vi "SBML_Functions.vi"(8 "error in (no error)":errorcluster, 11 "Input SBML File":string) -> (0 "error out":errorcluster, 1 "Fn Arg Cnt":string[](array[string]), 2 "Functions":string[][](table), 3 "FuncCnt":i32)   [LabVIEW 2014]
doc: "This VI extract the information of species present in SBML file. It takes the complete SBML file as input, and outputs: \nSp_Cnt --> How many species are there\nS_Id_Arr --> Array of species\nSp_Name --> Array containing the name of species\nSp_Init_Amnt --> Array containing the initial amount of species\n\nDesigned by HB\nhaba@dtu.dk"
panel:
  out "Math":string[](array[string])
  out "Name":string[](array[string])
  out "ID":string[](array[string])
  out "List of Functions":string
  # "Names"
  # "Initial Amount"
  # "ID"
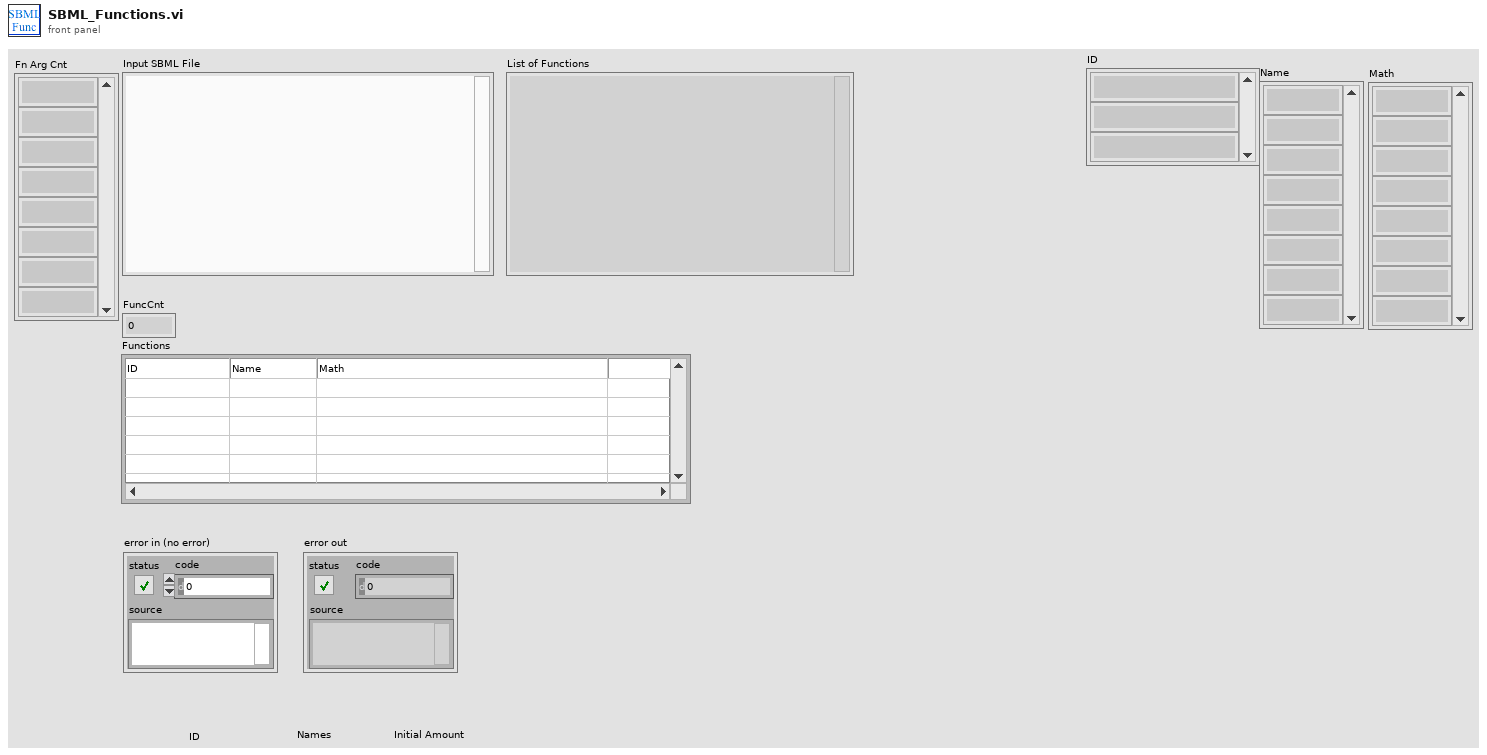
[diagram p1: front panel]
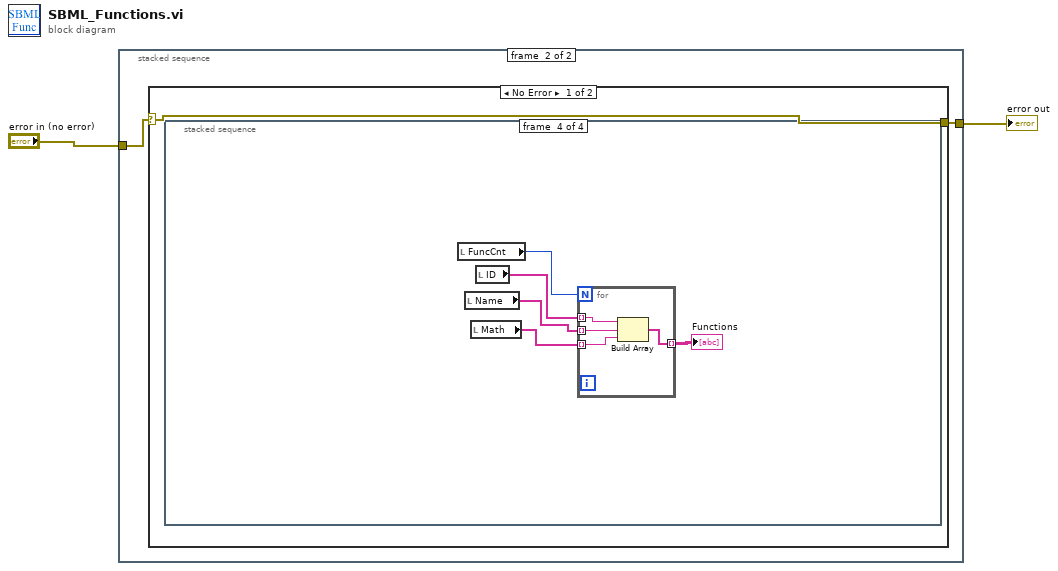
[diagram p0: block diagram]
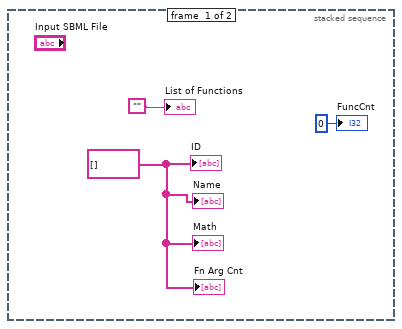
[diagram p2: hidden frame]
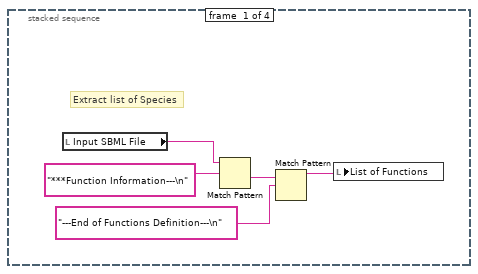
[diagram p3: hidden frame]
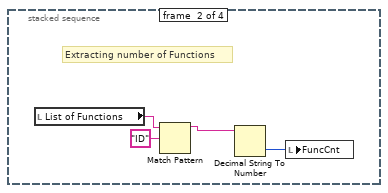
[diagram p4: hidden frame]
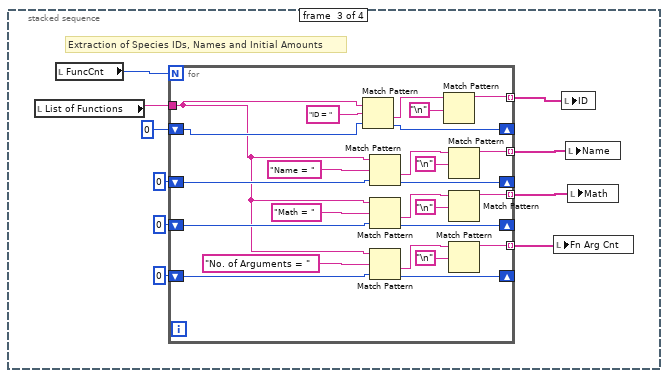
[diagram p5: hidden frame]
diagram:
  n1 = stacked-sequence {
    tunnel: "error in (no error)" -> [_ w6]
    tunnel: [_ w7] -> w1
    frame #0 {
      w3 = string[] [] ("Sp_Id_Arr")
      "List of Functions" <- "" ("Full SBML File")
      "FuncCnt" <- 0 ("Sp_cnt")
      "ID" <- w3
      "Name" <- w3
      "Math" <- w3
      "Fn Arg Cnt" <- w3
    }
    frame #1 {
      n2 = case shown="No Error" w6 {
        selector: w6 -> [w8 w62]
        tunnel: [w8 w62] -> w7
        frame No Error {
          n3 = stacked-sequence {
            frame #0 {
              # "Extract list of Species"
              n4 = local read "Input SBML File"() -> (w10:string)
              n5 = Match Pattern(string=w10, regular expression="***Function Information---\n") -> (after substring=w12:string)  [unwired: 1 in, 3 out]
              n6 = Match Pattern(string=w12, regular expression="---End of Functions Definition---\n") -> (before substring=w9:string)  [unwired: 1 in, 3 out]
              n7 = local write "List of Functions"(w9) -> ()
            }
            frame #1 {
              # "Extracting number of Functions"
              n8 = local read "List of Functions"() -> (w14:string)
              n9 = Match Pattern(string=w14, regular expression="ID") -> (before substring=w15:string)  [unwired: 1 in, 3 out]
              n10 = Decimal String To Number(string=w15) -> (number=w17:i32)  [unwired: 2 in, 1 out]
              n11 = local write "FuncCnt"(w17) -> ()
            }
            frame #2 {
              # "Extraction of Species IDs, Names and Initial Amounts"
              n12 = local read "List of Functions"() -> (w26:string)
              n13 = local read "FuncCnt"() -> (w25:i32)
              n14 = for {
                N: w25 -> [_]
                tunnel: w26 -> [w28]
                shift-right: [w41] -> _
                shift-left: 0 ("offset past match") -> [w42]
                tunnel: [w49] -> w24 mode=indexing
                shift-right: [w46] -> _
                shift-left: 0 ("offset past match") -> [w47]
                tunnel: [w48] -> w23 mode=indexing
                shift-right: [w37] -> _
                shift-left: 0 ("offset past match") -> [w36]
                tunnel: [w35] -> w20 mode=indexing
                shift-right: [w32] -> _
                shift-left: 0 ("offset past match") -> [w33]
                tunnel: [w34] -> w19 mode=indexing
                n15 = Match Pattern(string=w28, regular expression="ID = ", offset (0)=w42) -> (after substring=w50:string, offset past match=w41:i32)  [unwired: 2 out]
                n16 = Match Pattern(string=w28, regular expression="Name = ", offset (0)=w47) -> (after substring=w43:string, offset past match=w46:i32)  [unwired: 2 out]
                n17 = Match Pattern(string=w28, regular expression="Math = ", offset (0)=w36) -> (after substring=w40:string, offset past match=w37:i32)  [unwired: 2 out]
                n18 = Match Pattern(string=w28, regular expression="No. of Arguments = ", offset (0)=w33) -> (after substring=w29:string, offset past match=w32:i32)  [unwired: 2 out]
                n19 = Match Pattern(string=w50, regular expression="\n") -> (before substring=w49:string)  [unwired: 1 in, 3 out]
                n20 = Match Pattern(string=w43, regular expression="\n") -> (before substring=w48:string)  [unwired: 1 in, 3 out]
                n21 = Match Pattern(string=w40, regular expression="\n") -> (before substring=w35:string)  [unwired: 1 in, 3 out]
                n22 = Match Pattern(string=w29, regular expression="\n") -> (before substring=w34:string)  [unwired: 1 in, 3 out]
              }
              n23 = local write "Fn Arg Cnt"(w19) -> ()
              n24 = local write "ID"(w24) -> ()
              n25 = local write "Name"(w23) -> ()
              n26 = local write "Math"(w20) -> ()
            }
            frame #3 {
              n27 = local read "FuncCnt"() -> (w55:i32)
              n28 = local read "Name"() -> (w54:string[])
              n29 = local read "Math"() -> (w56:string[])
              n30 = local read "ID"() -> (w53:string[])
              n31 = for {
                N: w55 -> [_]
                tunnel: w53 -> [w61] mode=indexing
                tunnel: w54 -> [w60] mode=indexing
                tunnel: [w59] -> w57 mode=indexing
                tunnel: w56 -> [w58] mode=indexing
                n32 = Build Array(w61, w60, w58) -> (w59:string[])
              }
              "Functions" <- w57
            }
          }
        }
        frame Error {
        }
      }
    }
  }
  "error out" <- w1
